vi "Write Sizing.vi"(8 "error in (no error)":errorcluster, 10 "Sizing":T1, 11 "Splitter in":refnum<class "Splitter.lvclass">) -> (0 "error out":errorcluster, 3 "Splitter out":refnum<class "Splitter.lvclass">)   [LabVIEW 2015, in "Splitter.lvclass"]
uses:
  Splitter.lvclass
  Typedefs/Splitter Sizing--Enum.ctl
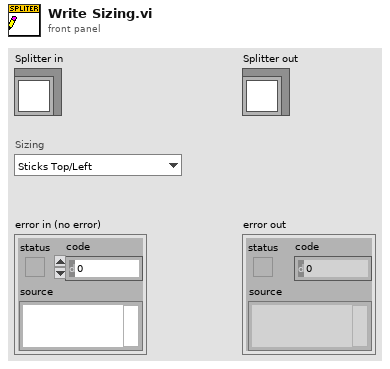
[diagram p1: front panel]
types:
  T1 = typedef "Splitter Sizing--Enum.ctl" = enum16{"Sticks Top/Left", "Sticks Bottom/Right", "Proportional"}
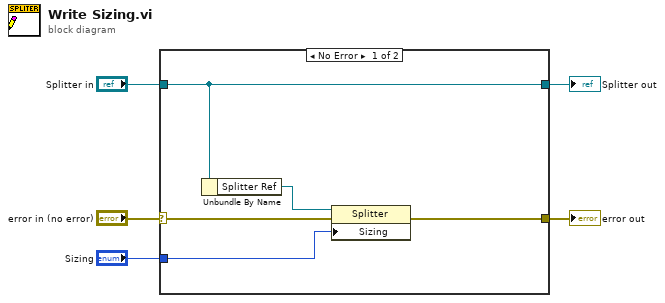
[diagram p0: block diagram]
diagram:
  n1 = case shown="No Error" "error in (no error)" {
    selector: "error in (no error)" -> [w10 w11]
    tunnel: [w9 w11] -> w4
    tunnel: [w8 w12] -> w2
    tunnel: "Splitter in" -> [w8 w12]
    tunnel: "Sizing" -> [w6 _]
    frame No Error {
      n2 = Unbundle By Name(w8) -> ("Splitter Ref"=w7:refnum<vi>)
      n3 = property class="Splitter"(reference=w7, error in=w10, "Sizing"=w6) -> (error out=w9:errorcluster)  [unwired: 1 out]
    }
    frame Error {
    }
  }
  "error out" <- w4
  "Splitter out" <- w2
